vi "Processing_SaveTXT.vi"(0 "Save?":bool, 1 "Piezo/nm":dbl[](array[numeric]), 2 "Bias/v":dbl[](array[numeric]), 3 "Log(G/G0)":dbl[](array[numeric]), 4 "File No":i32, 5 "Error In":errorcluster, 6 "Femto / V":dbl[](array[numeric]), 8 "File Path (use dialog)":path) -> (14 "File No Out":i32, 19 "Error Out":errorcluster)   [LabVIEW 2025]
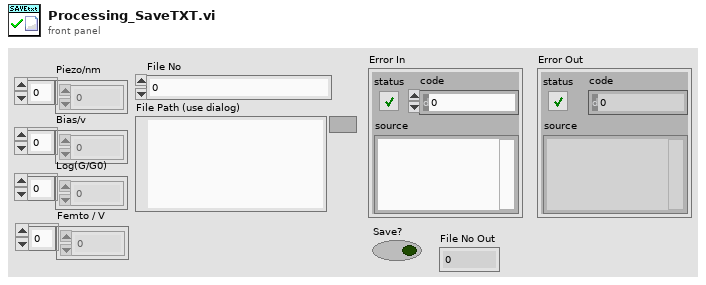
[diagram p1: front panel]
types:
  T1 = enum16{"open", "replace", "create", "open or create", "replace or create", "replace or create with confirmation"}
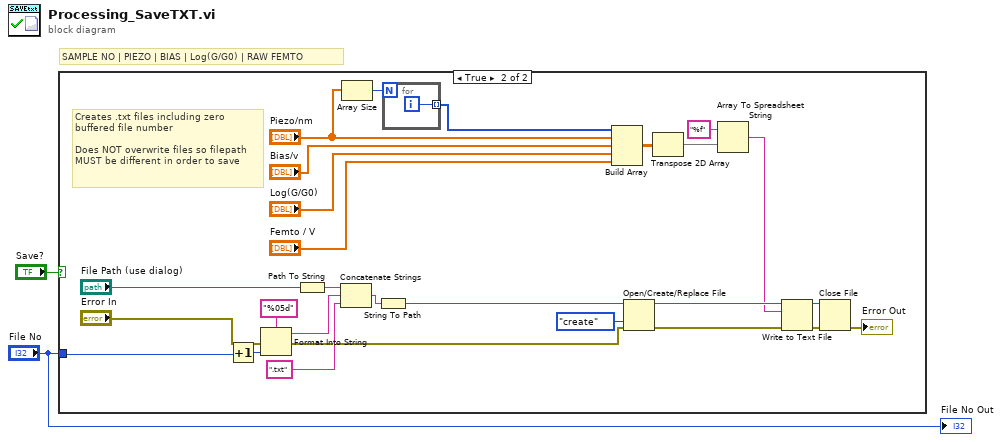
[diagram p0: block diagram]
diagram:
  # "SAMPLE NO | PIEZO | BIAS | Log(G/G0) | RAW FEMTO"
  n1 = case shown="True" "Save?" {
    tunnel: "File No" -> [_ w8]
    frame False {
      # "This is the water\nAnd this is the well.\nDrink full and descend.\nThe horse is the white of the eyes and dark within."
    }
    frame True {
      # "Creates .txt files including zero buffered file number\n\nDoes NOT overwrite files so filepath MUST be different in order to save"
      n2 = Increment(x=w8) -> (x+1=w21:i32)
      n3 = Format Into String(format string="%05d", error in="Error In", w21) -> (resulting string=w19:string, error out=w11:errorcluster)  [unwired: 1 in]
      n4 = Path To String(path="File Path (use dialog)") -> (string=w20:string)
      n5 = Concatenate Strings(w20, w19, ".txt" ("string")) -> (w23:string)
      n6 = Array Size(array="Piezo/nm") -> (size(s)=w7:i32)
      n7 = String To Path(string=w23) -> (path=w18:path)
      n8 = for {
        N: w7 -> [_]
        tunnel: [w30] -> w4 mode=indexing
        i -> [w30]
      }
      n9 = Build Array(w4, "Piezo/nm", "Bias/v", "Log(G/G0)", "Femto / V") -> (w13:dbl[][])
      n10 = Open/Create/Replace File(file path (use dialog)=w18, error in=w11, operation (0:open)=T1."create") -> (refnum out=w29:refnum<file>, error out=w28:errorcluster)  [unwired: 3 in, 1 out]
      n11 = Transpose 2D Array(2D array=w13) -> (transposed array=w12:dbl[][])
      n12 = Array To Spreadsheet String(array=w12, 3:"%f" ("format string")) -> (spreadsheet string=w16:string)  [unwired: 1 in]
      n13 = Write to Text File(file (use dialog)=w29, text=w16, error in=w28) -> (refnum out=w26:refnum<file>, error out=w27:errorcluster)  [unwired: 1 in, 1 out]
      n14 = Close File(refnum=w26, error in=w27) -> (error out=→"Error Out":errorcluster)  [unwired: 1 out]
    }
  }
  "File No Out" <- "File No"
